vi "rpm.vi"() -> ()   [LabVIEW 2019]
panel:
  out "Old_dTicks":i64
  out "deltaTicks":i64[](array[numeric])
  out "MaxDeltaNc":i64
  out "OldNc":i64
  out "MaxNc":i64
  out "Sigma deltaTicks":i64
  out "Multiplicant":dbl
  out "Max32":i64
  out "OldRPM":dbl
  out "comutations":i64
  out "prev_count":i64
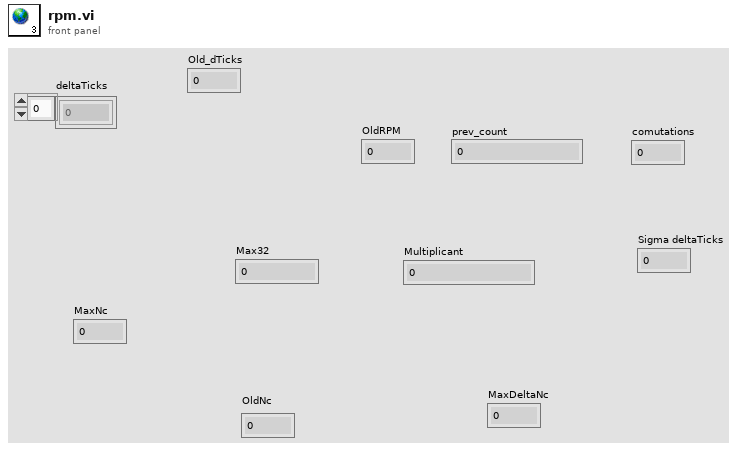
[diagram p1: front panel]
diagram:
